vi "OAT Get Even Angle Reference.vi"   [LabVIEW 2017, in "SoundVib_RefDataProcess.lvlib"]
doc: "Computes the even-angle reference of the <B>scaled signal [EU]</B>. The output reference is the even-angle spaced signal with a constant number of samples per revolution. Wire data to the <B>scaled signal [EU]</B> input to determine the polymorphic instance to use or manually select the instance."
uses:
  <vilib>/addons/Sound and Vibration/Order Analysis/Referece Data Processing/SoundVib_RefDataProcess.lvlib
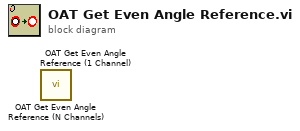
[diagram p0: block diagram]
diagram:
  n1 = call <vilib>:"OAT Get Even Angle Reference (N Channels).vi"() -> ()  [unwired: 13 in, 3 out]
  n2 = call <vilib>:"OAT Get Even Angle Reference (1 Channel).vi"() -> ()  [unwired: 13 in, 3 out]
